vi "Dip Stamp.vi"(8 "error in":errorcluster, 10 "Reservoir Number":i32, 11 "GrabberTool in":refnum<class "GrabberTool Class.lvclass">) -> (0 "error out":errorcluster, 3 "GrabberTool out":refnum<class "GrabberTool Class.lvclass">)   [LabVIEW 2017, in "GrabberTool Class.lvclass"]
uses:
  GrabberTool Class.lvclass
  Config Manager Class/Type Definitions/Named Position.ctl
  Config Manager Class/Type Definitions/Offset.ctl
  Config Manager Class/Type Definitions/Part Type.ctl
  WorkTable Class/WorkTable Class.lvclass
  Vec3d Class/Vec3d Class.lvclass
  Config Manager Class/Config Manager Class.lvclass
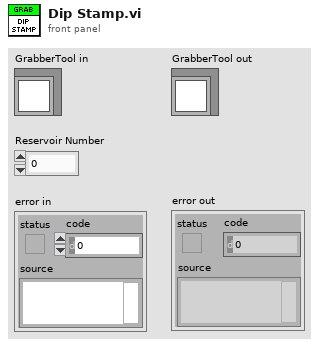
[diagram p1: front panel]
types:
  T1 = typedef "Part Type.ctl" = enum16{"BBM", "HDI", "BARE HDI", "GLUERESERVOIR", "STAMP_1", "STAMP_2", "STAMP_3", "STAMP_4", "STAMP_5", "STAMP_6", "STAMP_7", "STAMP_8", "WEIGHT_1", "WEIGHT_2", "WEIGHT_3", "WEIGHT_4", "WEIGHT_5", "WEIGHT_6", "WEIGHT_7", "WEIGHT_8", "WEIGHT_9", "WEIGHT_10", "WEIGHT_11", "WEIGHT_12", "WEIGHT_13", "WEIGHT_14", "WEIGHT_15", "WEIGHT_16", "PICKER_TOOL", "GRABER_TOOL"}
  T2 = typedef "Offset.ctl" = enum16{"tool_holder_offset"}
  T3 = typedef "Named Position.ctl" = enum16{"home", "module_chuck_0", "module_chuck_1", "module_chuck_2", "module_chuck_3", "module_chuck_4", "glue_reservoir_chuck", "stamp_tool_chuck", "weight_tool_chuck", "needle_calibration", "needle_calibration_camera", "tool_rack_pos_0_in", "tool_rack_pos_0_out", "tool_rack_pos_1_in", "tool_rack_pos_1_out", "tool_rack_pos_2_in", "tool_rack_pos_2_out", "front_load_position", "grabber_start_pos", "between_chuck_0_and_1", "between_chuck_2_and_3"}
  T4 = typedef "Worktable_Glue Reservoir.ctl" = cluster{"Glue Reservoir Slots":cluster{"Reservoir State":enum16{"Empty", "Full", "Used"}, "Center":refnum<class "Vec3d Class.lvclass">}[], "Vacuum Channel":i32}
  T5 = cluster{"Reservoir State":enum16{"Empty", "Full", "Used"}, "Center":refnum<class "Vec3d Class.lvclass">}[]
  T6 = cluster{"Reservoir State":enum16{"Empty", "Full", "Used"}, "Center":refnum<class "Vec3d Class.lvclass">}
  T7 = typedef "Stamp Type.ctl" = enum16{"Stamp 1", "Stamp 2", "Stamp 3", "Stamp 4", "Stamp 5", "Stamp 6", "Stamp 7", "Stamp 8"}
  T8 = typedef "Gluing Parameters.ctl" = cluster{"Safe Grabber Pickup":dbl, "Safe Grabber Lift":dbl, "Glue Resevoir Wait Time":dbl, "Glue BM Wait Time ":dbl, "Placed Weight X-Move":dbl}
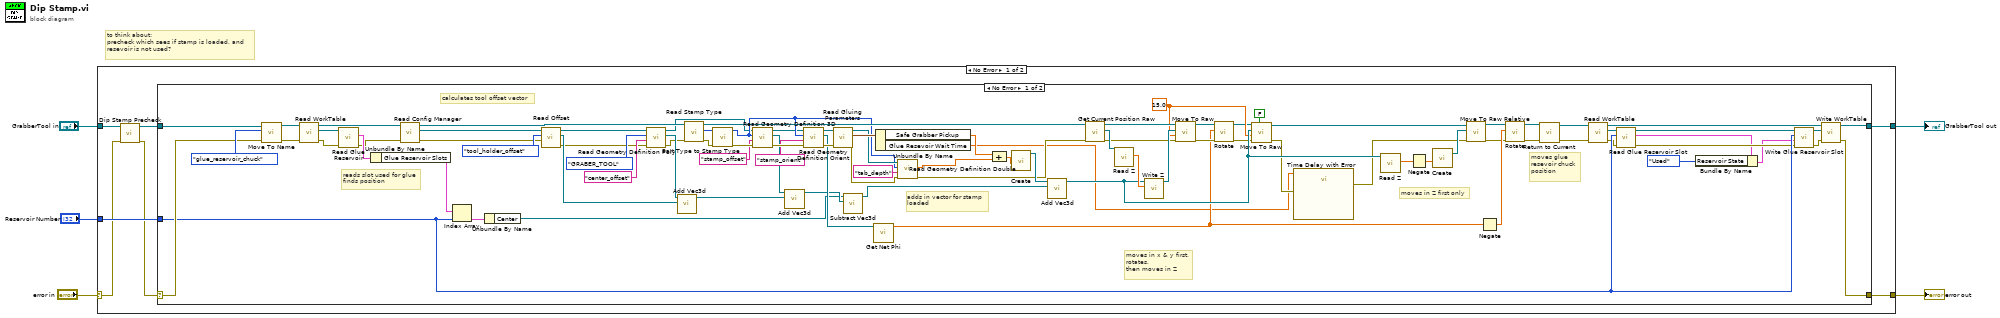
[diagram p0: block diagram]
diagram:
  # "to think about:\nprecheck which sees if stamp is loaded, and \nresevoir is not used?"
  n1 = case shown="No Error" "error in" {
    selector: "error in" -> [w7 w105]
    tunnel: [w12 w105] -> w5
    tunnel: "GrabberTool in" -> [w8 w106]
    tunnel: [w11 w106] -> w3
    tunnel: "Reservoir Number" -> [w10 _]
    frame No Error {
      n2 = call "Dip Stamp Precheck.vi"("error in (no error)"=w7, "GrabberTool Class in"=w8) -> ("error out"=w6:errorcluster, "GrabberTool Class out"=w9:refnum<class "GrabberTool Class.lvclass">)  [unwired: 8 in]
      n3 = case shown="No Error" w6 {
        selector: w6 -> [w77 w104]
        tunnel: [w51 w104] -> w12
        tunnel: [w56 w103] -> w11
        tunnel: w9 -> [w102 w103]
        tunnel: w10 -> [w57 _]
        frame No Error {
          w50 = 15.0 ("Speed")
          # "moves glue\nresevoir chuck\nposition"
          # "moves in Z first only"
          # "moves in x & y first,\nrotates,\nthen moves in Z"
          # "adds in vector for stamp\nloaded"
          # "reads slot used for glue\nfinds position"
          # "calculates tool offset vector"
          n4 = call-dynamic "Move To Name.vi"("error in"=w77, "Destination"=Named_Position."glue_reservoir_chuck", "Gantry in"=w102) -> ("error out"=w76:errorcluster, "Gantry out"=w100:refnum<class "GrabberTool Class.lvclass">)  [unwired: 7 in]
          n5 = call-dynamic "Read WorkTable.vi"("error in"=w76, "Gantry Class in"=w100) -> ("error out"=w75:errorcluster, "WorkTable Class.lvclass"=w89:refnum<class "WorkTable Class.lvclass">, "Gantry Class out"=w68:refnum<class "GrabberTool Class.lvclass">)  [unwired: 7 in]
          n6 = call-dynamic "Read Glue Reservoir.vi"("error in (no error)"=w75, "WorkTable Class in"=w89) -> ("error out"=w74:errorcluster, "Glue Reservoir"=w99:T4)  [unwired: 7 in, 1 out]
          n7 = Unbundle By Name(w99) -> ("Glue Reservoir Slots"=w98:T5)
          n8 = call-dynamic "Read Config Manager.vi"("error in"=w74, "Gantry in"=w68) -> ("error out"=w73:errorcluster, "Config Manager"=w92:refnum<class "Config Manager Class.lvclass">, "Gantry out"=w69:refnum<class "GrabberTool Class.lvclass">)  [unwired: 7 in]
          n9 = Index Array(array=w98, index=w57) -> (element=w97:T6)
          n10 = Unbundle By Name(w97) -> ("Center"=w20:refnum<class "Vec3d Class.lvclass">)
          n11 = call "Read Offset.vi"("error in"=w73, "Offset"=Offset."tool_holder_offset", "Config Manager in"=w92) -> ("error out"=w72:errorcluster, "Vec3d out"=w90:refnum<class "Vec3d Class.lvclass">, "Config Manager out"=w93:refnum<class "Config Manager Class.lvclass">)  [unwired: 6 in]
          n12 = call-poly "Read Geometry Definition Poly.vi"("error in"=w72, "Feature"="center_offset", "Part Type"=Part_Type."GRABER_TOOL", "Config Manager in"=w93) -> ("error out"=w66:errorcluster, "Feature Coordinates"=w91:refnum<class "Vec3d Class.lvclass">, "Config Manager out"=w40:refnum<class "Config Manager Class.lvclass">)  [unwired: 5 in]
          n13 = call-dynamic "Add Vec3d.vi"(10:"Vec3d Class in"=w90, 11:"Vec3d Class in"=w91) -> ("Vec3d Class out"=w23:refnum<class "Vec3d Class.lvclass">)  [unwired: 8 in, 1 out]
          n14 = call "Read Stamp Type.vi"("error in (no error)"=w66, "GrabberTool Class in"=w69) -> ("error out"=w65:errorcluster, "Stamp Type"=w67:T7, "GrabberTool Class out"=w70:refnum<class "GrabberTool Class.lvclass">)  [unwired: 7 in]
          n15 = call "Part Type to Stamp Type.vi"("error in"=w65, "Stamp Type"=w67) -> ("error out"=w41:errorcluster, "Part Type"=w46:T1)  [unwired: 8 in]
          n16 = call "Read Geometry Definition 3D.vi"("error in"=w41, "Feature"="stamp_offset", "Part Type"=w46, "Config Manager in"=w40) -> ("error out"=w42:errorcluster, "Feature Coordinates"=w37:refnum<class "Vec3d Class.lvclass">, "Config Manager out"=w45:refnum<class "Config Manager Class.lvclass">)  [unwired: 5 in]
          n17 = call-dynamic "Add Vec3d.vi"(10:"Vec3d Class in"=w23, 11:"Vec3d Class in"=w37) -> ("Vec3d Class out"=w21:refnum<class "Vec3d Class.lvclass">)  [unwired: 8 in, 1 out]
          n18 = call "Read Geometry Definition Orient.vi"("error in"=w42, "Feature"="stamp_orient", "Part Type"=w46, "Config Manager in"=w45) -> ("error out"=w43:errorcluster, "Orient3d out"=w36:refnum<class "Orient3d Class.lvclass">, "Config Manager out"=w44:refnum<class "Config Manager Class.lvclass">)  [unwired: 5 in]
          n19 = call "Read Gluing Parameters.vi"("error in (no error)"=w43, "Config Manager Class in"=w44) -> ("error out"=w71:errorcluster, "Gluing Parameters"=w88:T8, "Config Manager Class out"=w87:refnum<class "Config Manager Class.lvclass">)  [unwired: 7 in]
          n20 = call "Subtract Vec3d.vi"("Vec3d in 2"=w21, "Vec3d in 1"=w20) -> ("Vec3d Class out"=w22:refnum<class "Vec3d Class.lvclass">)  [unwired: 8 in, 1 out]
          n21 = call "Get Net Phi.vi"("Orient3d"=w36) -> ("phi(deg)"=w27:dbl)  [unwired: 8 in, 2 out]
          n22 = Unbundle By Name(w88) -> ("Safe Grabber Pickup"=w18:dbl, "Glue Resevoir Wait Time"=w14:dbl)
          n23 = call "Read Geometry Definition Double.vi"("error in"=w71, "Feature"="tab_depth", "Part Type"=w46, "Config Manager in"=w87) -> ("error out"=w64:errorcluster, "Geometry Definition"=w17:dbl)  [unwired: 5 in, 1 out]
          n24 = Compound Arithmetic op=ADD(w18, w17) -> (w19:dbl)
          n25 = call "Create.vi"("Z"=w19) -> ("Vec3d Class out"=w85:refnum<class "Vec3d Class.lvclass">)  [unwired: 9 in, 1 out]
          n26 = call-dynamic "Add Vec3d.vi"(10:"Vec3d Class in"=w22, 11:"Vec3d Class in"=w85) -> ("Vec3d Class out"=w80:refnum<class "Vec3d Class.lvclass">)  [unwired: 8 in, 1 out]
          n27 = call-dynamic "Get Current Position Raw.vi"("error in"=w64, "Gantry in"=w70) -> ("error out"=w63:errorcluster, "Vec3d Class out"=w84:refnum<class "Vec3d Class.lvclass">, "Gantry out"=w82:refnum<class "GrabberTool Class.lvclass">)  [unwired: 7 in]
          n28 = call-dynamic "Read Z.vi"("Vec3d Class in"=w84) -> ("Z"=w83:dbl)  [unwired: 8 in, 2 out]
          n29 = call-dynamic "Write Z.vi"("Z"=w83, "Vec3d Class in"=w80) -> ("Vec3d Class out"=w81:refnum<class "Vec3d Class.lvclass">)  [unwired: 8 in, 1 out]
          n30 = call-dynamic "Move To Raw.vi"("error in"=w63, "Speed"=w50, "Destination"=w81, "Gantry in"=w82) -> ("error out"=w32:errorcluster, "Gantry out"=w35:refnum<class "GrabberTool Class.lvclass">)  [unwired: 6 in]
          n31 = call-dynamic "Rotate.vi"("error in"=w32, "distance(deg)"=w27, "Gantry in"=w35) -> ("error out"=w33:errorcluster, "Gantry out"=w34:refnum<class "GrabberTool Class.lvclass">)  [unwired: 7 in]
          n32 = call-dynamic "Move To Raw.vi"("Wait?"=FALSE, "error in"=w33, "Speed"=w50, "Destination"=w80, "Gantry in"=w34) -> ("error out"=w15:errorcluster, "Gantry out"=w79:refnum<class "GrabberTool Class.lvclass">)  [unwired: 5 in]
          n33 = call "Time Delay with Error.vi"("error in (no error)"=w15, "Delay Time (s)"=w14) -> ("error out"=w13:errorcluster)  [unwired: 9 in]
          n34 = call-dynamic "Read Z.vi"("Vec3d Class in"=w80) -> ("Z"=w31:dbl)  [unwired: 8 in, 2 out]
          n35 = Negate(x=w31) -> (-x=w30:dbl)
          n36 = call "Create.vi"("Z"=w30) -> ("Vec3d Class out"=w78:refnum<class "Vec3d Class.lvclass">)  [unwired: 9 in, 1 out]
          n37 = call-dynamic "Move To Raw Relative.vi"("error in"=w13, "Delta"=w78, "Gantry in"=w79) -> ("error out"=w25:errorcluster, "Gantry out"=w29:refnum<class "GrabberTool Class.lvclass">)  [unwired: 7 in]
          n38 = Negate(x=w27) -> (-x=w26:dbl)
          n39 = call-dynamic "Rotate.vi"("error in"=w25, "distance(deg)"=w26, "Gantry in"=w29) -> ("error out"=w24:errorcluster, "Gantry out"=w28:refnum<class "GrabberTool Class.lvclass">)  [unwired: 7 in]
          n40 = call-dynamic "Return to Current.vi"("error in"=w24, "Gantry in"=w28) -> ("error out"=w55:errorcluster, "Gantry out"=w62:refnum<class "GrabberTool Class.lvclass">)  [unwired: 8 in]
          n41 = call-dynamic "Read WorkTable.vi"("error in"=w55, "Gantry Class in"=w62) -> ("error out"=w54:errorcluster, "WorkTable Class.lvclass"=w61:refnum<class "WorkTable Class.lvclass">, "Gantry Class out"=w59:refnum<class "GrabberTool Class.lvclass">)  [unwired: 7 in]
          n42 = call "Read Glue Reservoir Slot.vi"("error in (no error)"=w54, "index"=w57, "WorkTable Class in"=w61) -> ("error out"=w53:errorcluster, "Glue Resivoir Slot"=w49:T6, "WorkTable Class out"=w60:refnum<class "WorkTable Class.lvclass">)  [unwired: 6 in]
          n43 = Bundle By Name(cluster=w49, "Reservoir State"=enum16{"Empty", "Full", "Used"}."Used") -> (w48:T6)
          n44 = call "Write Glue Reservoir Slot.vi"("error in (no error)"=w53, "Glue Resivoir Slot"=w48, "index"=w57, "WorkTable Class in"=w60) -> ("error out"=w52:errorcluster, "WorkTable Class out"=w58:refnum<class "WorkTable Class.lvclass">)  [unwired: 6 in]
          n45 = call-dynamic "Write WorkTable.vi"("error in (no error)"=w52, "WorkTable Class.lvclass"=w58, "Gantry Class in"=w59) -> ("error out"=w51:errorcluster, "Gantry Class out"=w56:refnum<class "GrabberTool Class.lvclass">)  [unwired: 7 in]
        }
        frame Error {
        }
      }
    }
    frame Error {
    }
  }
  "error out" <- w5
  "GrabberTool out" <- w3
